vi "Create Folder or Check Folder already exit.vi"(6 "error in (no error)":errorcluster, 7 "Path In":path) -> (2 "error out":errorcluster, 3 "Path Out":path)   [LabVIEW 2017]
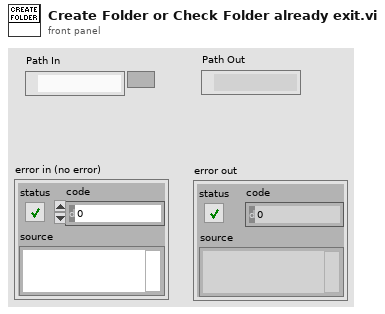
[diagram p1: front panel]
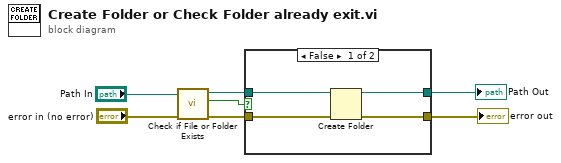
[diagram p0: block diagram]
diagram:
  n1 = call <vilib>:"Check if File or Folder Exists.vi"("error in (no error)"="error in (no error)", "path"="Path In") -> ("file or folder exists?"=w5:bool, "dup path"=w4:path)  [unwired: 7 in, 1 out]
  n2 = case shown="False" w5 {
    tunnel: w4 -> [w10 w12]
    tunnel: [w9 w12] -> w1
    tunnel: "error in (no error)" -> [w8 w11]
    tunnel: [w7 w11] -> w2
    frame False {
      n3 = Create Folder(path (use dialog)=w10, error in=w8) -> (created path=w9:path, error out=w7:errorcluster)  [unwired: 1 in, 1 out]
    }
    frame True {
    }
  }
  "error out" <- w2
  "Path Out" <- w1
